vi "Filter Enabled Lines Waveform.vi"(8 "error in (no error)":errorcluster, 10 "Pattern Digital Data":digitaldata, 11 "IO Lines Enable":T1={"Enable"=[FALSE, FALSE, FALSE, FALSE, FALSE, FALSE, FALSE, FALSE, FALSE, FALSE, FALSE, FALSE, FALSE, FALSE, FALSE, FALSE, FALSE, FALSE, FALSE, FALSE, FALSE, FALSE, FALSE, FALSE, FALSE, FALSE, FALSE, FALSE, FALSE, FALSE, FALSE, FALSE]}) -> (0 "error out":errorcluster, 2 "Digital Waveform":digitalwaveform(waveform)={"t0"=timestamp(0 s since 1904-01-01), "dt"=1.0, "Y"={"transitions"=[], "data"=[]}})   [LabVIEW 2016]
uses:
  Typedefs/IO Lines Enable.ctl
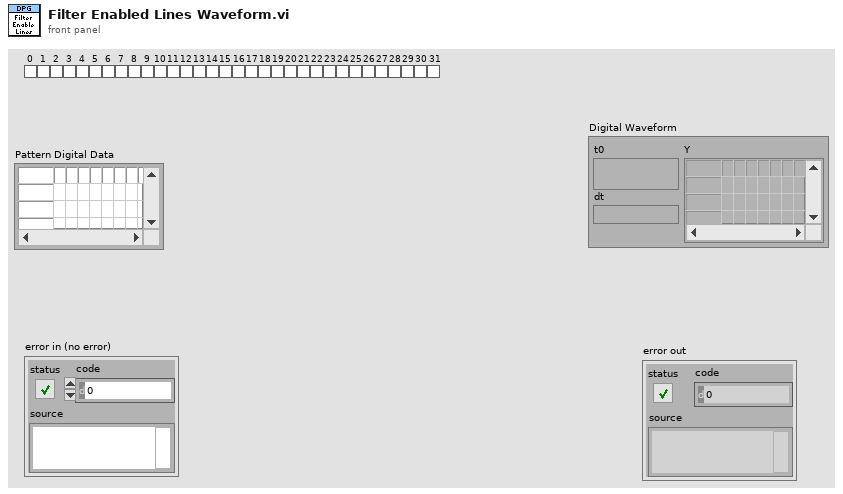
[diagram p1: front panel]
types:
  T1 = typedef "IO Lines Enable.ctl" = cluster{"Enable":bool[]}
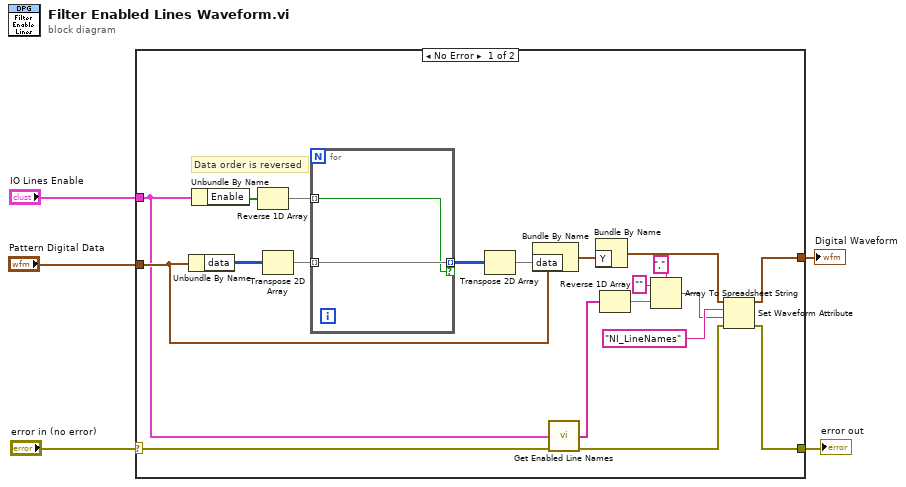
[diagram p0: block diagram]
diagram:
  n1 = case shown="No Error" "error in (no error)" {
    selector: "error in (no error)" -> [w17 w29]
    tunnel: "Pattern Digital Data" -> [w21 w28]
    tunnel: [w8 w29] -> w3
    tunnel: "IO Lines Enable" -> [w18 _]
    tunnel: [w6 w28] -> w1
    frame No Error {
      # "Data order is reversed"
      n2 = Unbundle By Name(w21) -> ("data"=w24:u8[][])
      n3 = Unbundle By Name(w18) -> ("Enable"=w25:bool[])
      n4 = Reverse 1D Array(array=w25) -> (reversed array=w23:bool[])
      n5 = Transpose 2D Array(2D array=w24) -> (transposed array=w22:u8[][])
      n6 = for {
        tunnel: w23 -> [w26] mode=indexing
        tunnel: w22 -> [w27] mode=indexing
        tunnel: [w27] -> w20 mode=indexing if=w26
      }
      n7 = Transpose 2D Array(2D array=w20) -> (transposed array=w19:u8[][])
      n8 = Bundle By Name(cluster=w21, "data"=w19) -> (w7:digitaldata)
      n9 = call "Get Enabled Line Names.vi"("IO Lines Enable"=w18, "error in (no error)"=w17) -> ("Enableld Line Names"=w10:string[], "error out"=w9:errorcluster)  [unwired: 12 in]
      n10 = Bundle By Name("Y"=w7) -> (w16:digitalwaveform)  [unwired: 1 in]
      n11 = Reverse 1D Array(array=w10) -> (reversed array=w11:string[])
      n12 = Array To Spreadsheet String(delimiter (Tab)=",", array=w11, 3:"" ("format string")) -> (spreadsheet string=w12:string)
      n13 = Set Waveform Attribute(4:w9, 5:w12, 6:"NI_LineNames" ("name"), 7:w16) -> (0:w8:errorcluster, 3:w6:digitalwaveform)  [unwired: 1 out]
    }
    frame Error {
    }
  }
  "error out" <- w3
  "Digital Waveform" <- w1
